vi "Lesson3 - Invoke Node demo.vi"() -> ()   [LabVIEW 2013]
panel:
  in  "Resinitialize to Default Value":bool
  in  "Stop Button 2":bool
  out "Tank 2":dbl(slide) scale=0.0..10.0
  in  "Vertical Fill Slide 2":dbl(slide) scale=0.0..10.0
  # "this is Property Node demonstration"
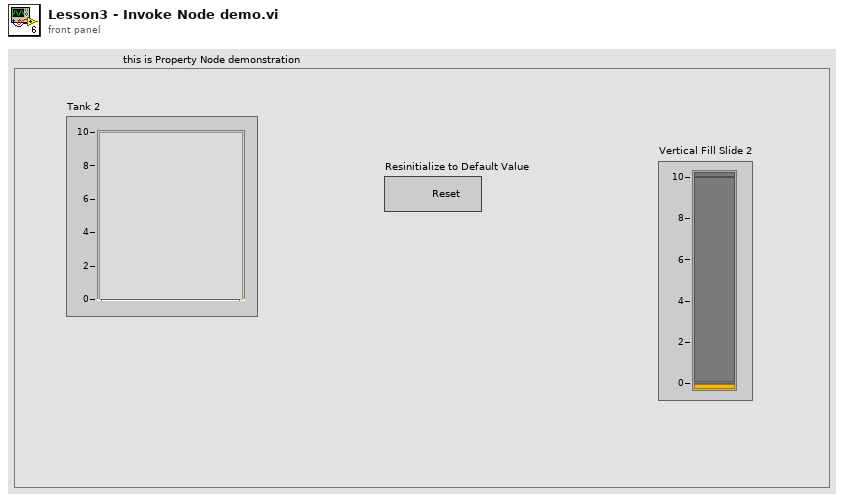
[diagram p1: front panel]
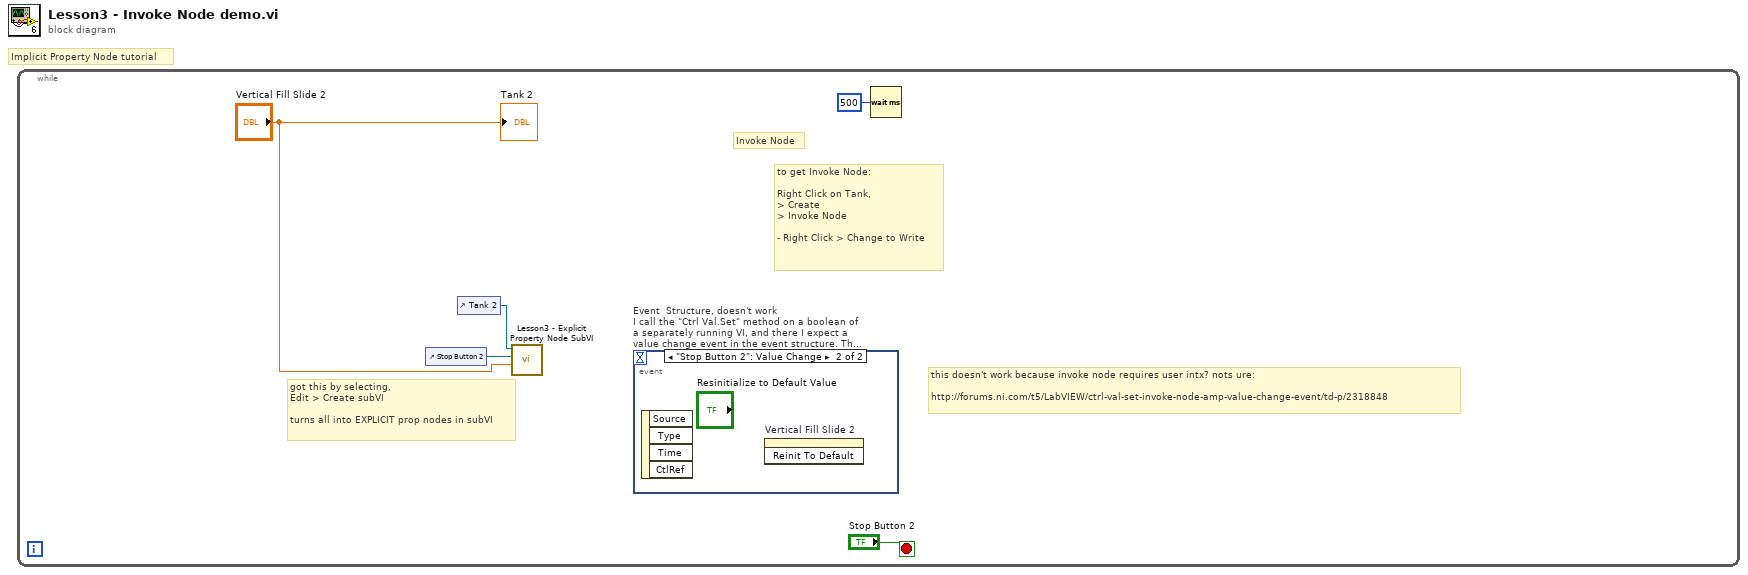
[diagram p0: block diagram]
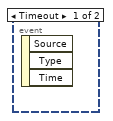
[diagram p2: hidden frame]
diagram:
  # "Implicit Property Node tutorial"
  n1 = while {
    stop <- "Stop Button 2" stop-if-true
    # "this doesn't work because invoke node requires user intx? nots ure:\n\nhttp://forums.ni.com/t5/LabVIEW/ctrl-val-set-invoke-node-amp-value-change-event/td-p/2318848"
    # "got this by selecting,\nEdit > Create subVI\n\nturns all into EXPLICIT prop nodes in subVI"
    # "to get Invoke Node:\n\nRight Click on Tank,\n> Create\n> Invoke Node\n\n- Right Click > Change to Write"
    # "Invoke Node"
    n2 = control-ref of="Stop Button 2"() -> (w1:refnum<vi>)
    n3 = control-ref of="Tank 2"() -> (w2:refnum<vi>)
    n4 = call "Lesson3 - Explicit Property Node SubVI.vi"("Vertical Fill Slide in"="Vertical Fill Slide 2", "Bool Refnum"=w1, "Slide in"=w2) -> ()  [unwired: 9 in]
    n5 = event "Event  Structure, doesn't work\nI call the \"Ctrl Val.Set\" method on a boolean of a separately running VI, and there I expect a value change event in the event structure. The value is changed, but no event is triggered. How can I enable a trigger?" shown="[1] \"Stop Button 2\": Value Change" {
      selector: _ -> [_ _]
      dyn-events: _ -> [_ _]
      timeout: _ -> [_ _]
      event Timeout {
        n6 = event-data() -> ()  [unwired: 1 in, 3 out]
      }
      event "Stop Button 2": Value Change {
        n7 = event-data() -> ()  [unwired: 1 in, 4 out]
        n8 = invoke on="Vertical Fill Slide 2" class="Slide (strict)" method="Reinit To Default"() -> ()  [unwired: 3 in, 3 out]
      }
    }
    n9 = Wait (ms)(milliseconds to wait=u32 500) -> ()  [unwired: 1 out]
    "Tank 2" <- "Vertical Fill Slide 2"
  }
